vi "Setup Calibration Board.vi"(8 "error in (no error)":errorcluster, 11 "App in":refnum<class "App.lvclass">) -> (0 "error out":errorcluster, 3 "App out":refnum<class "App.lvclass">)   [LabVIEW 2020, in "AR Example.lvlib" / "App.lvclass"]
uses:
  App.lvclass
  App.lvclass/App.ctl
  g_ar_toolkit.image/New Image (Greyscale).vi
  g_ar_toolkit.image/Interpolation Mode.ctl
  g_ar_toolkit.common/Image Size (Integer).ctl
  g_ar_toolkit.common/Object Point (Float).ctl
  g_ar_toolkit.feature_detection/Apriltag Detector/Detector Settings.ctl
  g_ar_toolkit.image/Resize (Greyscale).vi
  g_ar_toolkit.image/Copy Array to Image (Greyscale).vi
  g_ar_toolkit.feature_detection/AprilTagStandard41h12IDList.vi
  g_ar_toolkit.feature_detection/Apriltag Detector/Create (Tag36h11).vi
  g_ar_toolkit.feature_detection/GenerateApriltag36h11.vi
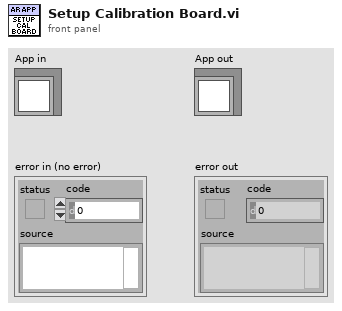
[diagram p1: front panel]
types:
  T1 = typedef "g_ar_toolkit.feature_detection.lvlib/AprilTag Detector.lvclass/Detector Settings.ctl" = cluster{"Refine Edges (Default: True)":bool, "Threads (Default: 1)":u8, "Decimate (Default: 1)":sgl, "Blur (Default: 0)":sgl, "Bits (Default: 2)":u8}
  T2 = typedef "g_ar_toolkit.common.lvlib/Object Point (Float).ctl" = cluster{"x":dbl, "y":dbl, "z":dbl}
  T3 = typedef "g_ar_toolkit.common.lvlib/Image Size (Integer).ctl" = cluster{"Width":u16, "Height":u16}
  T4 = typedef "g_ar_toolkit.image.lvlib/Interpolation Mode.ctl" = enum8{"NEAREST", "LINEAR", "CUBIC", "AREA", "LANCZOS", "LINEAR_EXACT", "NEAREST_EXACT", "MAX"}
  T5 = typedef "g_ar_toolkit.image.lvlib/Greyscale Image.ctl" = refnum<data-value>
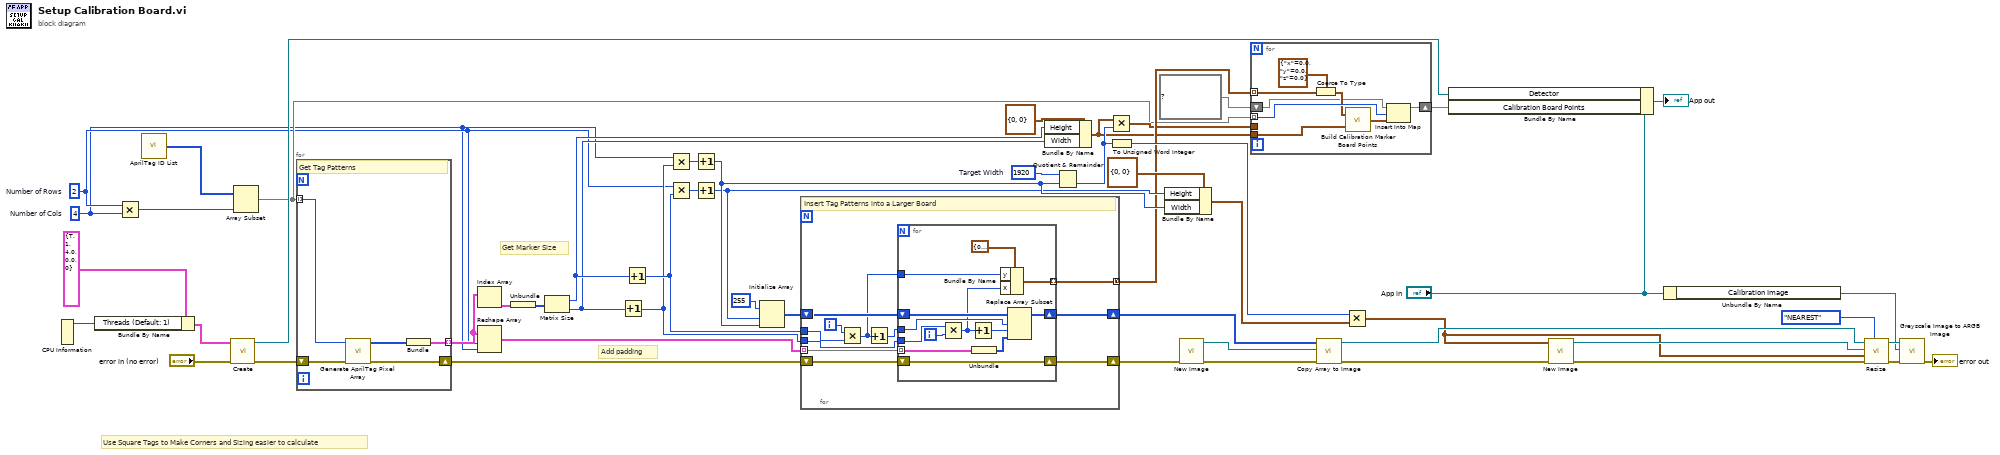
[diagram p0: block diagram]
diagram:
  w33 = 1920  # Target Width
  w3 = 4  # Number of Cols
  w4 = 2  # Number of Rows
  # "Use Square Tags to Make Corners and Sizing easier to calculate"
  # "Add padding"
  # "Get Marker Size"
  n1 = CPU Information() -> (4:w11:i32)  [unwired: 3 out]
  n2 = Bundle By Name(cluster=T1 {"Refine Edges (Default: True)"=TRUE, "Threads (Default: 1)"=1, "Decimate (Default: 1)"=4.0, "Blur (Default: 0)"=0.0, "Bits (Default: 2)"=0} ("Detector Settings"), "Threads (Default: 1)"=w11) -> (w12:T1)
  n3 = Multiply(x=w4, y=w3) -> (x*y=w8:i32)
  n4 = call-poly "AprilTag ID List.vi"() -> ("Tag IDs"=w50:i32[])
  n5 = call-poly "Create.vi"("error in (no error)"="error in (no error)", "Detector Settings"=w12) -> ("error out"=w14:errorcluster, "New Apriltag Detector"=w10:refnum<class "AprilTag Detector.lvclass">)  [unwired: 8 in]
  n6 = Array Subset(array=w50, length=w8) -> (w6:i32[])  [unwired: 1 in]
  n7 = for {
    tunnel: [w54] -> w5 mode=indexing
    shift-right: [w58] -> w49
    shift-left: w14 -> [w57]
    tunnel: w6 -> [w56] mode=indexing
    # "Get Tag Patterns"
    n8 = call-poly "Generate AprilTag Pixel Array.vi"("error in (no error)"=w57, "ID"=w56) -> ("error out"=w58:errorcluster, "Tag Pixel Array"=w55:u8[][])  [unwired: 8 in]
    n9 = Bundle("Tag Pixel Array"=w55) -> (w54:cluster{"Tag Pixel Array":u8[][]})  [unwired: 1 in]
  }
  n10 = Index Array(array=w5) -> (element=w7:cluster{"Tag Pixel Array":u8[][]})  [unwired: 1 in]
  n11 = Reshape Array(w5, w4, w3) -> (w1:cluster{"Tag Pixel Array":u8[][]}[][])
  n12 = Unbundle(w7) -> ("Tag Pixel Array"=w2:u8[][])
  n13 = Matrix Size(0:w2) -> (1:w29:i32, 2:w28:i32)
  n14 = Increment(x=w28) -> (x+1=w34:i32)
  n15 = Increment(x=w29) -> (x+1=w35:i32)
  n16 = Multiply(x=w3, y=w34) -> (x*y=w53:i32)
  n17 = Multiply(x=w4, y=w35) -> (x*y=w52:i32)
  n18 = Increment(x=w53) -> (x+1=w31:i32)
  n19 = Increment(x=w52) -> (x+1=w30:i32)
  n20 = Initialize Array(u8 255, w30, w31) -> (w48:u8[][])
  n21 = for {
    shift-right: [w68] -> w26
    shift-left: w49 -> [w69]
    shift-right: [w66] -> w43
    shift-left: w48 -> [w67]
    tunnel: w34 -> [w63]
    tunnel: w35 -> [w62]
    tunnel: [w61] -> w25 mode=concatenating
    tunnel: w1 -> [w59] mode=indexing
    i -> [w65]
    # "Insert Tag Patterns into a Larger Board"
    n22 = Multiply(x=w65, y=w62) -> (x*y=w60:i32)
    n23 = Increment(x=w60) -> (x+1=w64:i32)
    n24 = for {
      shift-right: [w82] -> w68
      shift-left: w69 -> [w82]
      shift-right: [w80] -> w66
      shift-left: w67 -> [w81]
      tunnel: w64 -> [w77]
      tunnel: w63 -> [w78]
      tunnel: [w74] -> w61 mode=indexing
      tunnel: w60 -> [w73]
      tunnel: w59 -> [w71] mode=indexing
      i -> [w79]
      n25 = Multiply(x=w78, y=w79) -> (x*y=w72:i32)
      n26 = Increment(x=w72) -> (x+1=w76:i32)
      n27 = Unbundle(w71) -> ("Tag Pixel Array"=w70:u8[][])
      n28 = Bundle By Name(cluster=cluster{"x":i32, "y":i32, "z":i32} {"x"=0, "y"=0, "z"=0} ("32bit integer"), "y"=w73, "x"=w72) -> (w74:cluster{"x":i32, "y":i32, "z":i32})
      n29 = Replace Array Subset(array=w81, new element=w70, index (row)=w77, index (col)=w76) -> (w80:u8[][])
    }
  }
  n30 = Bundle By Name(cluster=T3 {"Width"=0, "Height"=0} ("32bit integer"), "Height"=w29, "Width"=w28) -> (w9:T3)
  n31 = Quotient & Remainder(x=w33, y=w31) -> (floor(x/y)=w27:i32)  [unwired: 1 out]
  n32 = Multiply(x=w9, y=w27) -> (x*y=w24:cluster{"Width":i32, "Height":i32})
  n33 = To Unsigned Word Integer(number=w27) -> (unsigned 16bit integer=w32:u16)
  n34 = Bundle By Name(cluster=T3 {"Width"=0, "Height"=0} ("New Image Size"), "Height"=w30, "Width"=w31) -> (w41:T3)
  n35 = call-poly "New Image.vi"("error in (no error)"=w26) -> ("error out"=w40:errorcluster, "New Greyscale Image"=w47:T5)  [unwired: 9 in]
  n36 = for {
    tunnel: w6 -> [w90] mode=indexing
    tunnel: w25 -> [w89] mode=indexing
    tunnel: w24 -> [_]
    shift-right: [w86] -> w16
    shift-left: map{i32, T2[]} {} ("Size: 0") -> [w85]
    tunnel: w9 -> [w83]
    n37 = Coerce To Type(0:w89, 1:T2 {"x"=0.0, "y"=0.0, "z"=0.0}) -> (2:w88:T2)
    n38 = call "Build Calibration Marker Board Points.vi"("Marker Size"=w83, "Top Left Point"=w88) -> ("Marker Corners - AprilTag Detector Order"=w87:T2[])
    n39 = Insert Into Map(map in=w85, key=w90, value=w87) -> (map out=w86:map{i32, T2[]})  [unwired: 2 out]
  }
  n40 = call-poly "Copy Array to Image.vi"("error in (no error)"=w40, "Greyscale Destination Image"=w47, "U8 Greyscale Data"=w43) -> ("error out"=w39:errorcluster, "Greyscale Destination Image (duplicate)"=w45:T5)  [unwired: 7 in]
  n41 = Multiply(x=w32, y=w41) -> (x*y=w36:T3)
  n42 = Bundle By Name(cluster="App in", "Detector"=w10, "Calibration Board Points"=w16) -> (→"App out":refnum<class "App.lvclass">)
  n43 = call-poly "New Image.vi"("error in (no error)"=w39, "Preallocated Image Size (Default 0,0)"=w36) -> ("error out"=w37:errorcluster, "New Greyscale Image"=w38:T5)  [unwired: 8 in]
  n44 = Unbundle By Name("App in") -> ("Calibration Image"=w19:refnum<data-value>)
  n45 = call-poly "Resize.vi"("Interpolation Mode (Default: CUBIC)"=Interpolation_Mode."NEAREST", "error in (no error)"=w37, "New Image Size"=w36, "Greyscale Destination Image"=w38, "Greyscale Source Image"=w45) -> ("error out"=w21:errorcluster, "Greyscale Destination Image (duplicate)"=w20:T5)  [unwired: 5 in]
  n46 = call "Greyscale Image to ARGB Image.vi"("error in (no error)"=w21, "ARGB Image Destination"=w19, "Greyscale Image Source"=w20) -> ("error out"=→"error out":errorcluster)  [unwired: 7 in, 1 out]
